vi "SMTP Email Detect Code Type.vi"(11 "text in":string) -> (2 "code type":T1(ring))   [LabVIEW 2011, in "NewNI_SMTPEmail.lvlib"]
doc: "This VI detects type of Japanese encoding. Its primary purpose is to determine whether the input is of type Shift-JIS (SJIS), EUC, EUCORSJIS (indeterminate), or other."
uses:
  NewNI_SMTPEmail.lvlib
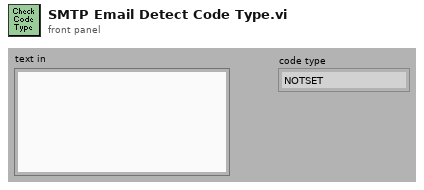
[diagram p1: front panel]
types:
  T1 = enum16{"NOTSET", "NEW", "OLD", "NEC", "EUC", "SJIS", "EUCORSJIS", "ASCII"}
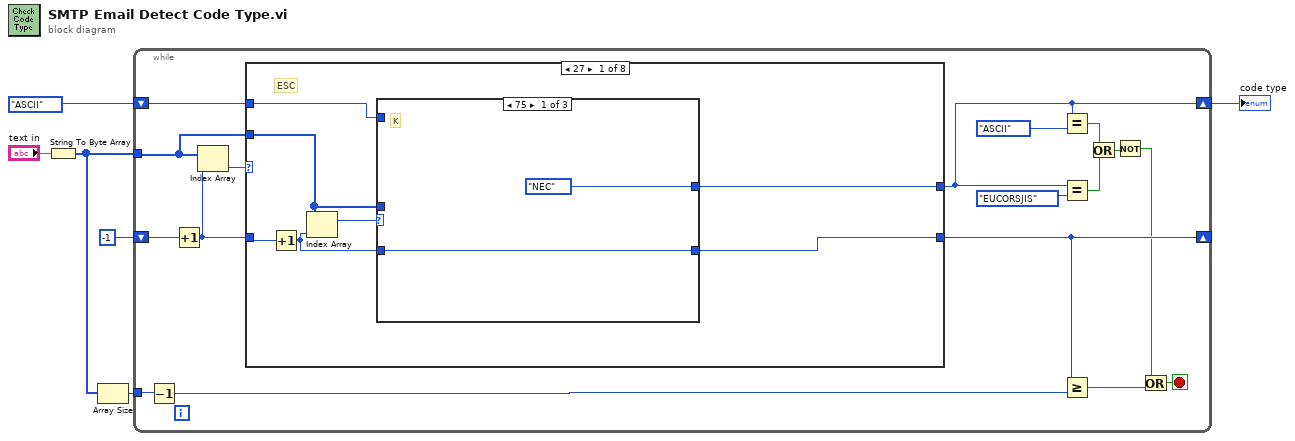
[diagram p0: block diagram]
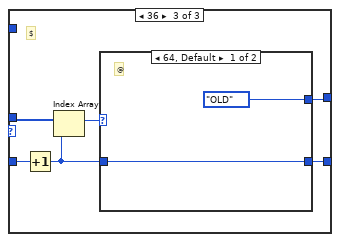
[diagram p3: hidden frame]
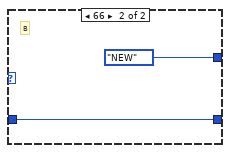
[diagram p4: hidden frame]
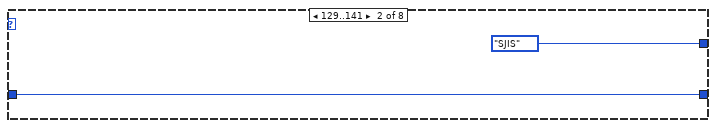
[diagram p5: hidden frame]
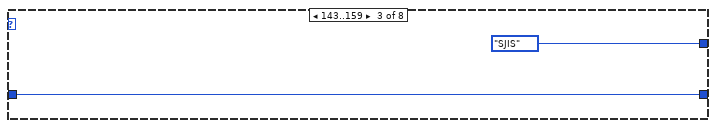
[diagram p6: hidden frame]
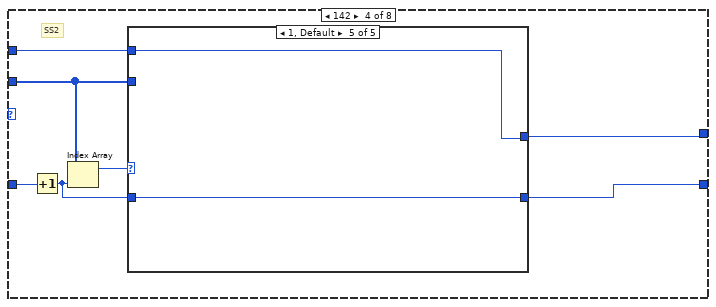
[diagram p7: hidden frame]
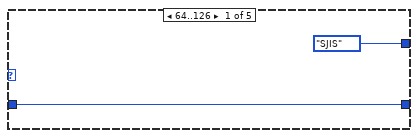
[diagram p8: hidden frame]
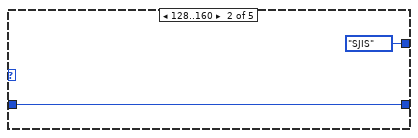
[diagram p9: hidden frame]
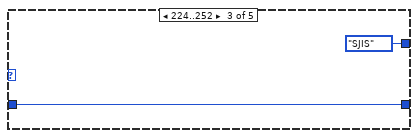
[diagram p10: hidden frame]
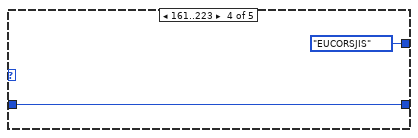
[diagram p11: hidden frame]
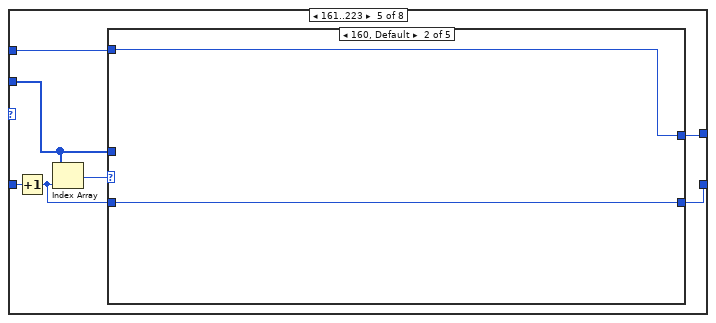
[diagram p12: hidden frame]
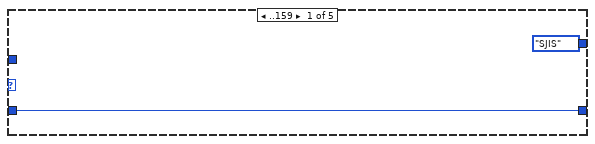
[diagram p13: hidden frame]
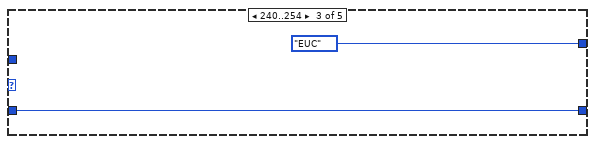
[diagram p14: hidden frame]
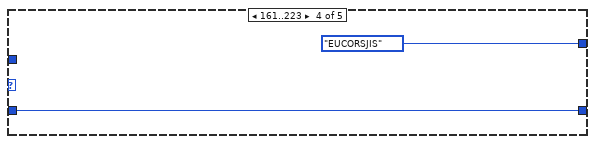
[diagram p15: hidden frame]
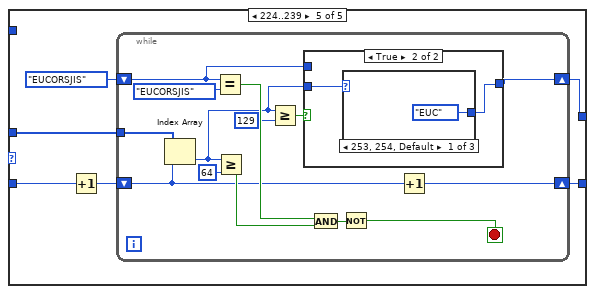
[diagram p16: hidden frame]
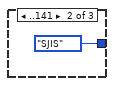
[diagram p18: hidden frame]
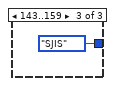
[diagram p19: hidden frame]
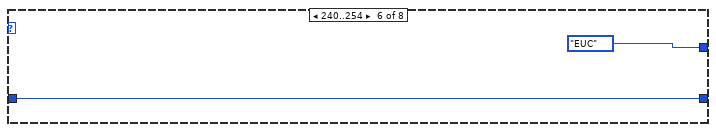
[diagram p20: hidden frame]
diagram:
  n1 = String To Byte Array(string="text in") -> (unsigned byte array=w2:u8[])
  n2 = Array Size(array=w2) -> (size(s)=w1:i32)
  n3 = while {
    shift-right: [w14] -> w3
    shift-left: T1."ASCII" ("Enum") -> [w19]
    tunnel: w2 -> [w21]
    shift-right: [w18] -> _
    shift-left: -1 -> [w22]
    tunnel: w1 -> [w17]
    stop <- w7 stop-if-true
    n4 = Decrement(x=w17) -> (x-1=w16:i32)
    n5 = Increment(x=w22) -> (x+1=w20:i32)
    n6 = Index Array(array=w21, index=w20) -> (element=w23:u8)
    n7 = case shown="27" w23 {
      tunnel: w19 -> [w24 _ _ w53 w72 _ w109 w127]
      tunnel: [w29 T1."SJIS" ("Enum") T1."SJIS" ("Enum") w54 w70 T1."EUC" ("Enum") w112 w127] -> w14
      tunnel: w20 -> [w28 w45 w47 w52 w68 w107 w115 w126]
      tunnel: w21 -> [w26 _ _ w50 w67 _ w114 _]
      tunnel: [w25 w45 w47 w49 w66 w107 w111 w126] -> w18
      frame 27 {
        # "ESC"
        n8 = Increment(x=w28) -> (x+1=w30:i32)
        n9 = Index Array(array=w26, index=w30) -> (element=w27:u8)
        n10 = case shown="75" w27 {
          tunnel: [T1."NEC" ("Enum") w34 w37] -> w29
          tunnel: w26 -> [_ _ w40]
          tunnel: w30 -> [w31 w33 w39]
          tunnel: [w31 w33 w35] -> w25
          tunnel: w24 -> [_ w34 _]
          frame 75 {
            # "K"
          }
          frame 76, Default {
          }
          frame 36 {
            # "$"
            n11 = Increment(x=w39) -> (x+1=w36:i32)
            n12 = Index Array(array=w40, index=w36) -> (element=w38:u8)
            n13 = case shown="64, Default" w38 {
              tunnel: [T1."OLD" ("Enum") T1."NEW" ("Enum")] -> w37
              tunnel: w36 -> [w41 w43]
              tunnel: [w41 w43] -> w35
              frame 64, Default {
                # "@"
              }
              frame 66 {
                # "B"
              }
            }
          }
        }
      }
      frame 129..141 {
      }
      frame 143..159 {
      }
      frame 142 {
        # "SS2"
        n14 = Increment(x=w52) -> (x+1=w51:i32)
        n15 = Index Array(array=w50, index=w51) -> (element=w55:u8)
        n16 = case shown="1, Default" w55 {
          tunnel: [T1."SJIS" ("Enum") T1."SJIS" ("Enum") T1."SJIS" ("Enum") T1."EUCORSJIS" ("Enum") w65] -> w54
          tunnel: w53 -> [_ _ _ _ w65]
          tunnel: w51 -> [w56 w58 w60 w62 w64]
          tunnel: w50 -> [_ _ _ _ _]
          tunnel: [w56 w58 w60 w62 w64] -> w49
          frame 64..126 {
          }
          frame 128..160 {
          }
          frame 224..252 {
          }
          frame 161..223 {
          }
          frame 1, Default {
          }
        }
      }
      frame 161..223 {
        n17 = Increment(x=w68) -> (x+1=w69:i32)
        n18 = Index Array(array=w67, index=w69) -> (element=w71:u8)
        n19 = case shown="160, Default" w71 {
          tunnel: w72 -> [_ w76 _ _ _]
          tunnel: [T1."SJIS" ("Enum") w76 T1."EUC" ("Enum") T1."EUCORSJIS" ("Enum") w82] -> w70
          tunnel: w69 -> [w73 w75 w77 w79 w85]
          tunnel: w67 -> [_ _ _ _ w86]
          tunnel: [w73 w75 w77 w79 w83] -> w66
          frame ..159 {
          }
          frame 160, Default {
          }
          frame 240..254 {
          }
          frame 161..223 {
          }
          frame 224..239 {
            n20 = Increment(x=w85) -> (x+1=w84:i32)
            n21 = while {
              tunnel: w86 -> [w100]
              shift-right: [w92] -> w83
              shift-left: w84 -> [w93]
              shift-right: [w87] -> w82
              shift-left: T1."EUCORSJIS" ("y") -> [w88]
              stop <- w94 stop-if-true
              n22 = Index Array(array=w100, index=w93) -> (element=w89:u8)
              n23 = Equal?(x=w88, y=T1."EUCORSJIS") -> (x = y?=w97:bool)
              n24 = Greater Or Equal?(x=w89, y=u8 64) -> (x >= y?=w96:bool)
              n25 = Greater Or Equal?(x=w89, y=u8 129) -> (x >= y?=w90:bool)
              n26 = case shown="True" w90 {
                tunnel: w89 -> [_ w103]
                tunnel: w88 -> [w101 _]
                tunnel: [w101 w102] -> w87
                frame False {
                }
                frame True {
                  n27 = case shown="253, 254, Default" w103 {
                    tunnel: [T1."EUC" ("y") T1."SJIS" ("y") T1."SJIS" ("y")] -> w102
                    frame 253, 254, Default {
                    }
                    frame ..141 {
                    }
                    frame 143..159 {
                    }
                  }
                }
              }
              n28 = And(x=w97, y=w96) -> (x .and. y?=w95:bool)
              n29 = Not(x=w95) -> (.not. x?=w94:bool)
              n30 = Increment(x=w93) -> (x+1=w92:i32)
            }
          }
        }
      }
      frame 240..254 {
      }
      frame 224..239 {
        n31 = Increment(x=w115) -> (x+1=w110:i32)
        n32 = Index Array(array=w114, index=w110) -> (element=w113:u8)
        n33 = case shown="127, Default" w113 {
          tunnel: [T1."SJIS" ("Enum") T1."SJIS" ("Enum") T1."EUC" ("Enum") T1."EUCORSJIS" ("Enum") w125] -> w112
          tunnel: [w116 w118 w120 w122 w124] -> w111
          tunnel: w110 -> [w116 w118 w120 w122 w124]
          tunnel: w109 -> [_ _ _ _ w125]
          frame 64..126 {
          }
          frame 128..160 {
          }
          frame 253, 254 {
          }
          frame 161..252 {
          }
          frame 127, Default {
          }
        }
      }
      frame 1, Default {
      }
    }
    n34 = Equal?(x=w14, y=T1."ASCII") -> (x = y?=w11:bool)
    n35 = Equal?(x=w14, y=T1."EUCORSJIS") -> (x = y?=w12:bool)
    n36 = Greater Or Equal?(x=w18, y=w16) -> (x >= y?=w8:bool)
    n37 = Or(x=w11, y=w12) -> (x .or. y?=w10:bool)
    n38 = Not(x=w10) -> (.not. x?=w9:bool)
    n39 = Or(x=w9, y=w8) -> (x .or. y?=w7:bool)
  }
  "code type" <- w3
